vi "load.vi"(8 "error in (no error)":errorcluster, 10 "functional":refnum<user-event>, 11 "interface_light in":refnum<class "light.lvclass">=refnum) -> (0 "error out":errorcluster, 3 "interface_light out":refnum<class "light.lvclass">)   [LabVIEW 2015, in "example_01.lvlib" / "light.lvclass"]
uses:
  light.lvclass
  functional/public/_controls/event_functional.ctl
  functional/public/_controls/event_functional_command.ctl
  functional/functional.lvlib
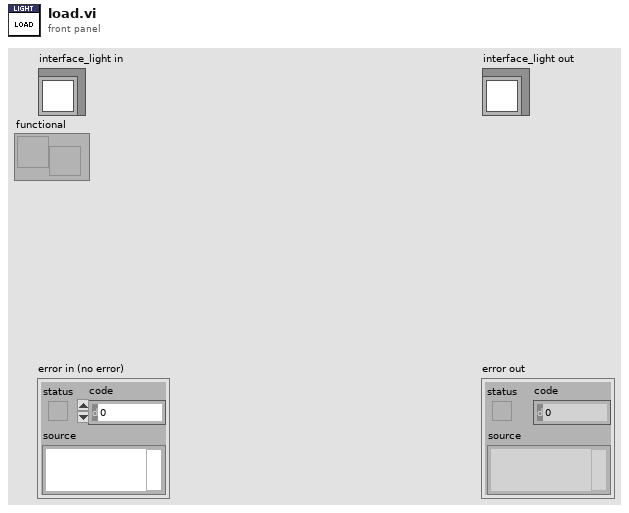
[diagram p1: front panel]
types:
  T1 = enum32{"Invalid", "Standard", "Closed", "Hidden", "Minimized", "Maximized"}
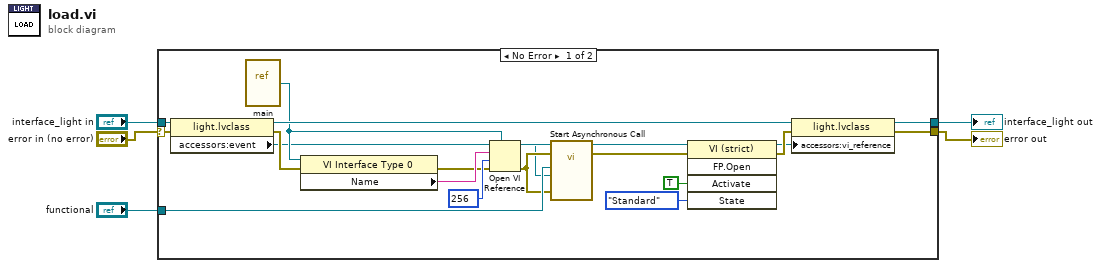
[diagram p0: block diagram]
diagram:
  n1 = case shown="No Error" "error in (no error)" {
    selector: "error in (no error)" -> [w9 w27]
    tunnel: [w11 w27] -> w2
    tunnel: [w15 w26] -> w1
    tunnel: "interface_light in" -> [w13 w26]
    tunnel: "functional" -> [w25 _]
    frame No Error {
      n2 = property class="light.lvclass"(reference=w13, error in=w9) -> (reference out=w12:refnum<class "light.lvclass">, error out=w8:errorcluster, "accessors:event"=w6:refnum<user-event>)
      n3 = vi-ref "main.vi"() -> (w7:refnum<vi>)
      n4 = property class="VI Interface Type 0"(reference=w7, error in=w8) -> (error out=w20:errorcluster, "Name"=w21:string)  [unwired: 1 out]
      n5 = Open VI Reference(type specifier VI Refnum (for type only)=w7, vi path=w21, options=256, error in (no error)=w20) -> (vi reference=w22:refnum<vi>, error out=w23:errorcluster)  [unwired: 2 in]
      n6 = call-by-ref "Start Asynchronous Call"(reference=w22, error in=w23, 8:"error in (no error)"=w23, "event"=w6, "functional"=w25) -> (reference out=w19:refnum<vi>, error out=w18:errorcluster)  [unwired: 8 in, 1 out]
      n7 = invoke class="VI (strict)" method="FP.Open"(reference=w19, error in=w18, "Activate"=TRUE ("Activate?"), "State"=T1."Standard") -> (reference out=w10:refnum<vi>, error out=w14:errorcluster)  [unwired: 1 in, 3 out]
      n8 = property class="light.lvclass"(reference=w12, error in=w14, "accessors:vi_reference"=w10) -> (reference out=w15:refnum<class "light.lvclass">, error out=w11:errorcluster)
    }
    frame Error {
    }
  }
  "error out" <- w2
  "interface_light out" <- w1
